vi "DropVI_SimpleReconnectingPublisher.vi"() -> ()   [LabVIEW 2013, in "MQTT Client.lvlib"]
uses:
  MQTT Client.lvlib
  <vilib>/LabVIEW Open Source Project/MQTT Connection/MQTT_Connection/Connection/Connection.lvclass
  Client class/Client.lvclass/Client.ctl
  <vilib>/LabVIEW Open Source Project/MQTT Connection/MQTT_Base/Base Class/MQTT_Base.lvclass/MQTT_Base.ctl
  <vilib>/LabVIEW Open Source Project/MQTT Control Packets/Control Packets/PUBLISH/PUBLISH.lvclass
  Client class/Client.lvclass
  <vilib>/LabVIEW Open Source Project/MQTT Connection/MQTT_Base/Base Class/MQTT_Base.lvclass
panel:
  out "Connected":bool
  out "last error":errorcluster
  out "Waveform Chart":dbl(graph)
  out "Published":bool
  in  "Stop Client":bool
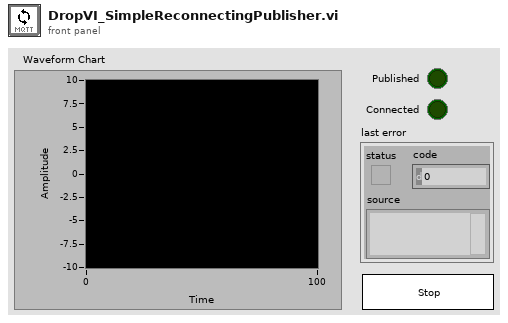
[diagram p1: front panel]
types:
  T1 = typedef "MQTT Client.lvlib/Client.lvclass/Public Events -- cluster.ctl" = cluster{"Connection Status":refnum<user-event>, "Connected":refnum<user-event>, "Application Message":refnum<user-event>}
  T2 = typedef "MQTT Base.lvlib/MQTT_Base.lvclass/Public Events -- cluster.ctl" = cluster{"Stop Event":refnum<user-event>, "Error Event":refnum<user-event>, "Inbound Message":refnum<user-event>}
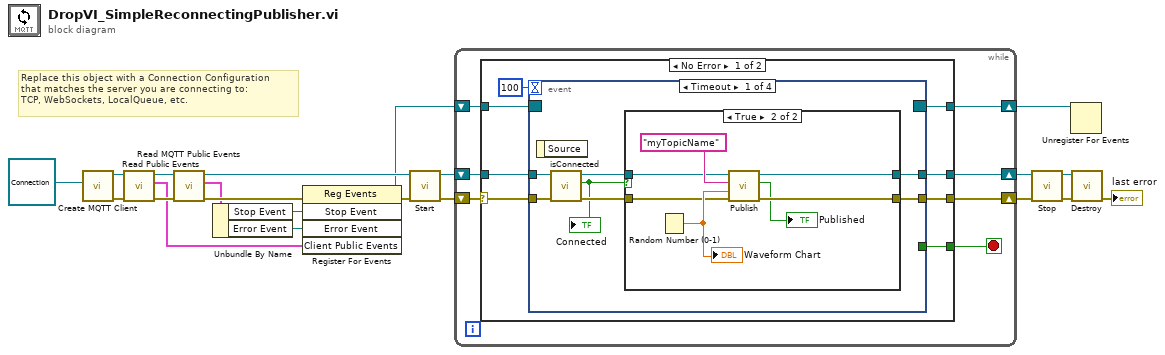
[diagram p0: block diagram]
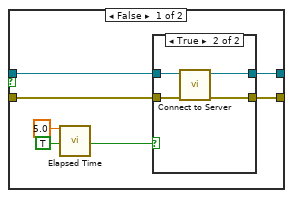
[diagram p2: hidden frame]
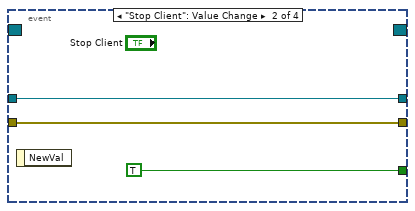
[diagram p4: hidden frame]
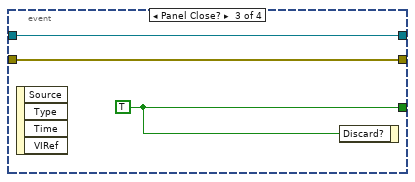
[diagram p5: hidden frame]
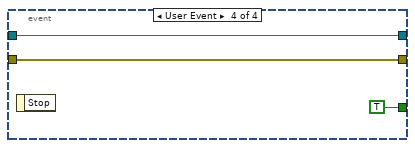
[diagram p6: hidden frame]
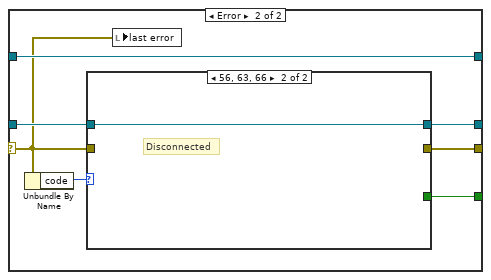
[diagram p7: hidden frame]
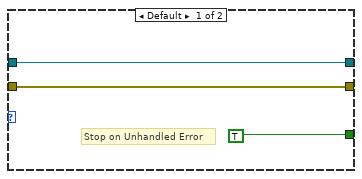
[diagram p8: hidden frame]
diagram:
  # "Replace this object with a Connection Configuration\nthat matches the server you are connecting to:\nTCP, WebSockets, LocalQueue, etc."
  n1 = call "Create MQTT Client.vi"("Connection Configuration"=refnum<class "Connection.lvclass"> refnum) -> ("error out"=w19:errorcluster, "Client out"=w21:refnum<class "Client.lvclass">)  [unwired: 9 in]
  n2 = call "Read Public Events.vi"("error in (no error)"=w19, "Client in"=w21) -> ("error out"=w18:errorcluster, "Client Public Events"=w16:T1, "Client out"=w20:refnum<class "Client.lvclass">)  [unwired: 7 in]
  n3 = call <vilib>:"Read MQTT Public Events.vi"("error in (no error)"=w18, "MQTT_Base in"=w20) -> ("error out"=w17:errorcluster, "MQTT Public Events"=w9:T2, "MQTT_Base out"=w14:refnum<class "Client.lvclass">)  [unwired: 7 in]
  n4 = Unbundle By Name(w9) -> ("Stop Event"=w11:refnum<user-event>, "Error Event"=w10:refnum<user-event>)
  n5 = register-events(error in=w17, w11, w10, w16) -> (reference out=w13:refnum<event-registration>, error out=w15:errorcluster)  [unwired: 1 in]
  n6 = call <vilib>:"Start.vi"("error in (no error)"=w15, "MQTT_Base in"=w14) -> ("error out"=w2:errorcluster, "MQTT_Base out"=w3:refnum<class "Client.lvclass">)  [unwired: 7 in, 1 out]
  n7 = while {
    shift-right: [w27] -> w12
    shift-left: w13 -> [w28]
    shift-right: [w24] -> w6
    shift-left: w3 -> [w25]
    shift-right: [w26] -> w4
    shift-left: w2 -> [w22]
    stop <- w23 stop-if-true
    n8 = case shown="No Error" w22 {
      selector: w22 -> [w29 w73]
      tunnel: w28 -> [w36 w79]
      tunnel: [w35 w79] -> w27
      tunnel: [w34 w75] -> w26
      tunnel: w25 -> [w32 w77]
      tunnel: [w31 w76] -> w24
      tunnel: [w30 w74] -> w23
      frame No Error {
        n9 = event shown="[0] Timeout" {
          selector: w36 -> [_ _ _ _]
          dyn-events: [_ _ _ _] -> w35
          timeout: 100 -> [_ _ _ _]
          tunnel: w29 -> [w39 w65 w67 w72]
          tunnel: [w42 w65 w67 w72] -> w34
          tunnel: [_ TRUE w69 TRUE] -> w30
          tunnel: w32 -> [w41 w66 w68 w70]
          tunnel: [w43 w66 w68 w70] -> w31
          event Timeout {
            n10 = event-data() -> ()  [unwired: 1 in, 1 out]
            n11 = call "isConnected.vi"("error in (no error)"=w39, "Client in"=w41) -> ("error out"=w38:errorcluster, "connected"=w37:bool, "Client out"=w40:refnum<class "Client.lvclass">)  [unwired: 7 in]
            "Connected" <- w37
            n12 = case shown="True" w37 {
              tunnel: [w49 w62] -> w43
              tunnel: [w47 w61] -> w42
              tunnel: w40 -> [w50 w58]
              tunnel: w38 -> [w48 w57]
              frame False {
                n13 = call "Elapsed Time"("Time Target (s)"=5.0, "Auto Reset"=TRUE) -> ("Time has Elapsed"=w46:bool)  [unwired: 10 in, 7 out]
                n14 = case shown="True" w46 {
                  tunnel: w50 -> [w52 w56]
                  tunnel: [w52 w55] -> w49
                  tunnel: w48 -> [w51 w54]
                  tunnel: [w51 w53] -> w47
                  frame False {
                  }
                  frame True {
                    n15 = call "Connect to Server.vi"("error in (no error)"=w54, "Client in"=w56) -> ("error out"=w53:errorcluster, "Client out"=w55:refnum<class "Client.lvclass">)  [unwired: 6 in, 2 out]
                  }
                }
              }
              frame True {
                n16 = Random Number (0-1)() -> (number: 0 to 1=w59:dbl)
                "Waveform Chart" <- w59
                n17 = call "Publish.vi"("error in (no error)"=w57, "Payload"=w59, "Topic Name (empty: Payload name)"="myTopicName", "Client in"=w58) -> ("error out"=w61:errorcluster, "Published"=→"Published":bool, "Client out"=w62:refnum<class "Client.lvclass">)  [unwired: 5 in]
              }
            }
          }
          event "Stop Client": Value Change {
            n18 = event-data() -> ()  [unwired: 1 in, 1 out]
          }
          event Panel Close? {
            w69 = TRUE
            n19 = event-data() -> ()  [unwired: 1 in, 4 out]
            n20 = event-data("Discard?"=w69) -> ()  [unwired: 1 in, 1 out]
          }
          event User Event {
            n21 = event-data() -> ()  [unwired: 1 in, 1 out]
          }
        }
      }
      frame Error {
        n22 = Unbundle By Name(w73) -> ("code"=w78:i32)
        n23 = case shown="56, 63, 66" w78 {
          tunnel: w77 -> [w82 w83]
          tunnel: [w82 w83] -> w76
          tunnel: w73 -> [w81 _]
          tunnel: [w81 _] -> w75
          tunnel: [TRUE _] -> w74
          frame Default {
            # "Stop on Unhandled Error"
          }
          frame 56, 63, 66 {
            # "Disconnected"
          }
        }
        n24 = local write "last error"(w73) -> ()
      }
    }
  }
  n25 = call <vilib>:"Stop.vi"("error in (no error)"=w4, "MQTT_Base in"=w6) -> ("error out"=w5:errorcluster, "MQTT_Base out"=w7:refnum<class "Client.lvclass">)  [unwired: 7 in, 1 out]
  n26 = Unregister For Events(event registration refnum=w12) -> ()  [unwired: 1 in, 1 out]
  n27 = call <vilib>:"Destroy.vi"("error in (no error)"=w5, "MQTT_Base in"=w7) -> ("error out"=→"last error":errorcluster)  [unwired: 8 in, 1 out]
